vi "C867_Macro.vi"(8 "error in":errorcluster caption="entrée d'erreur") -> (0 "error out":errorcluster caption="sortie d'erreur")   [LabVIEW 2026]
uses:
  Controls/TypeDef_FGV.ctl
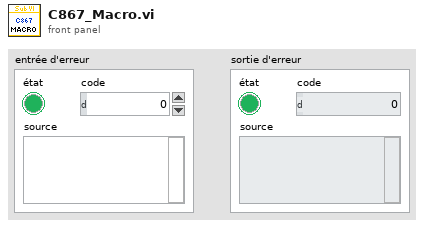
[diagram p1: front panel]
types:
  T1 = typedef "TypeDef_FGV.ctl" = enum16{"Initialize", "Write", "Read"}
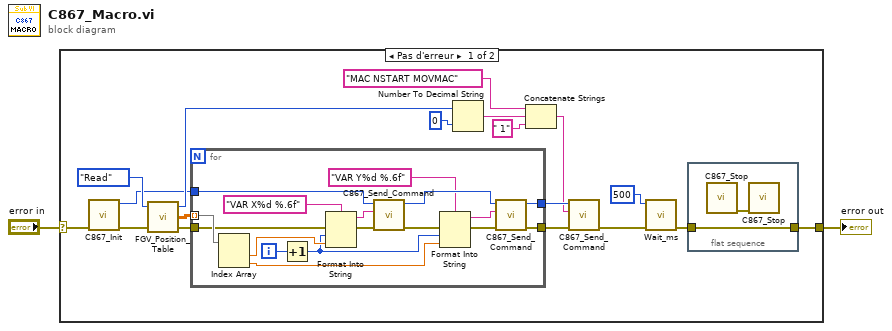
[diagram p0: block diagram]
diagram:
  n1 = case shown="Pas d'erreur" "error in" {
    selector: "error in" -> [w11 w40]
    tunnel: [w3 w40] -> w1
    frame No Error {
      n2 = call "C867_Init.vi"("error in"=w11) -> ("error out"=w10:errorcluster, "ID"=w9:i32)  [unwired: 9 in]
      n3 = call "FGV_Position_Table.vi"("error in"=w10, "Action"=TypeDef_FGV."Read") -> ("error out"=w20:errorcluster, "Position table"=w19:dbl[][], "N pos"=w15:i32)  [unwired: 1 in]
      n4 = for {
        tunnel: w19 -> [w39] mode=indexing
        tunnel: w20 -> [w38]
        tunnel: w9 -> [w31]
        tunnel: [w24] -> w8
        tunnel: [w23] -> w6
        i -> [w28]
        n5 = Index Array(array=w39) -> (element #1=w29:dbl, element #2=w26:dbl)  [unwired: 2 in]
        n6 = Increment(x=w28) -> (x+1=w25:i32)
        n7 = Format Into String(format string="VAR X%d %.6f" ("chaîne initiale"), error in=w38, w25, w29) -> (resulting string=w36:string, error out=w35:errorcluster)  [unwired: 1 in]
        n8 = call "C867_Send_Command.vi"("entrée d'erreur (pas d'erreur)"=w35, "szCommand"=w36, "ID en entrée"=w31) -> ("sortie d'erreur"=w32:errorcluster, "ID en sortie"=w30:i32)  [unwired: 5 in, 2 out]
        n9 = Format Into String(format string="VAR Y%d %.6f" ("chaîne initiale"), error in=w32, w25, w26) -> (resulting string=w33:string, error out=w34:errorcluster)  [unwired: 1 in]
        n10 = call "C867_Send_Command.vi"("entrée d'erreur (pas d'erreur)"=w34, "szCommand"=w33, "ID en entrée"=w30) -> ("sortie d'erreur"=w24:errorcluster, "ID en sortie"=w23:i32)  [unwired: 5 in, 2 out]
      }
      n11 = Number To Decimal String(number=w15, width (-)=i16 0 ("largeur (-)")) -> (decimal integer string=w14:string)
      n12 = Concatenate Strings("MAC NSTART MOVMAC", w14, " 1" ("chaîne")) -> (w5:string)
      n13 = call "C867_Send_Command.vi"("entrée d'erreur (pas d'erreur)"=w8, "szCommand"=w5, "ID en entrée"=w6) -> ("sortie d'erreur"=w7:errorcluster)  [unwired: 5 in, 3 out]
      n14 = call "Wait_ms.vi"("error in (no error)"=w7, "milliseconds to wait"=u32 500) -> ("error out"=w4:errorcluster)  [unwired: 9 in]
      n15 = flat-sequence {
        tunnel: [w21] -> w3
        tunnel: w4 -> [w21]
        frame #0 {
          n16 = call "C867_Stop.vi"() -> ("error out"=w22:errorcluster)  [unwired: 11 in]
          n17 = call "C867_Stop.vi"("error in"=w22) -> ()  [unwired: 10 in, 1 out]
        }
      }
    }
    frame Error {
    }
  }
  "error out" <- w1
